vi "VI Tree.vi"   [LabVIEW 2020, in "QDict.lvlib"]
doc: "Developed by Kevin Thompson\nkevin@thompsonengineering.net\n\nCopyright 2021\nThompson Engineering, LLC"
uses:
  QDict.lvlib
panel:
  # "SEE BLOCK DIAGRAM FOR MEMBER VIs"
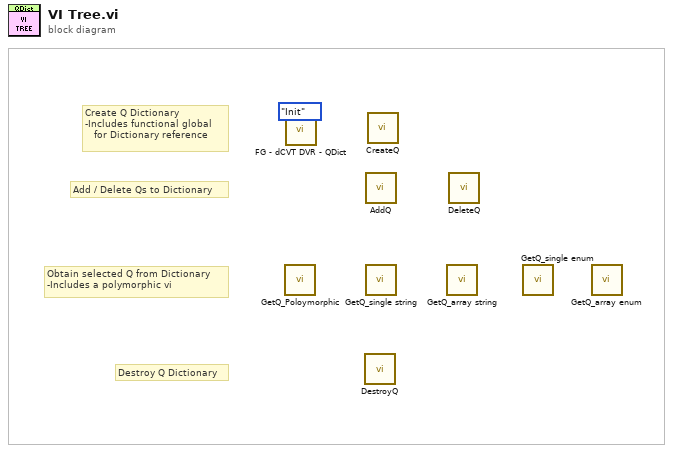
[diagram p0: block diagram]
diagram:
  # "Destroy Q Dictionary"
  # "Obtain selected Q from Dictionary\n-Includes a polymorphic vi"
  # "Add / Delete Qs to Dictionary"
  # "Create Q Dictionary\n-Includes functional global\n   for Dictionary reference"
  n1 = call-poly "GetQ_Poloymorphic.vi"() -> ()  [unwired: 9 in, 3 out]
  n2 = call "FG - dCVT DVR - QDict.vi"("Action (Get)"=enum16{"Init", "Get", "Set"}."Init") -> ()  [unwired: 8 in, 2 out]
  n3 = call "DestroyQ.vi"() -> ()  [unwired: 11 in, 1 out]
  n4 = call "AddQ.vi"() -> ()  [unwired: 10 in, 2 out]
  n5 = call "GetQ_single string.vi"() -> ()  [unwired: 9 in, 3 out]
  n6 = call "CreateQ.vi"() -> ()  [unwired: 10 in, 2 out]
  n7 = call "GetQ_array string.vi"() -> ()  [unwired: 9 in, 3 out]
  n8 = call "DeleteQ.vi"() -> ()  [unwired: 10 in, 2 out]
  n9 = call "GetQ_single enum.vi"() -> ()  [unwired: 9 in, 3 out]
  n10 = call "GetQ_array enum.vi"() -> ()  [unwired: 9 in, 3 out]
